vi "align_arrays.vi"(9 "IS_FRACTION":bool, 10 "Array 2":u8[](array[numeric]), 11 "Array":u8[](array[numeric])) -> (2 "Array 4":u8[](array[numeric]), 3 "Array 3":u8[](array[numeric]))   [LabVIEW 2025]
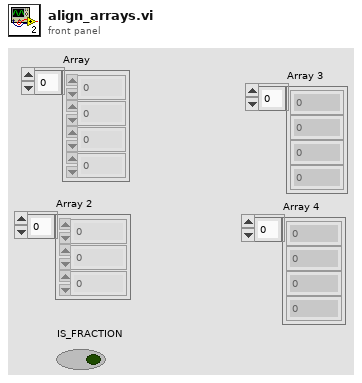
[diagram p1: front panel]
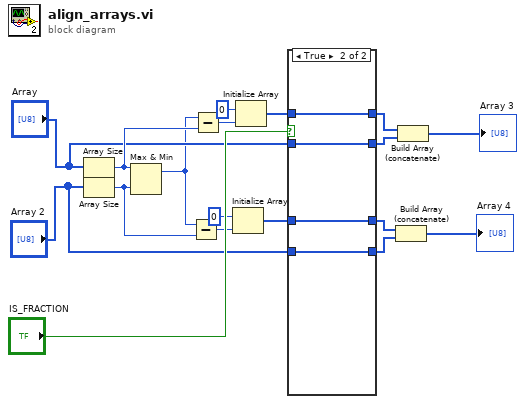
[diagram p0: block diagram]
diagram:
  n1 = Array Size(array="Array") -> (size(s)=w18:i32)
  n2 = Array Size(array="Array 2") -> (size(s)=w7:i32)
  n3 = Max & Min(x=w18, y=w7) -> (max(x,y)=w8:i32)  [unwired: 1 out]
  n4 = Subtract(x=w8, y=w7) -> (x-y=w6:i32)
  n5 = Subtract(x=w8, y=w18) -> (x-y=w17:i32)
  n6 = Initialize Array(u8 0 ("element"), w6) -> (w5:u8[])
  n7 = Initialize Array(u8 0 ("element"), w17) -> (w14:u8[])
  n8 = case shown="True" "IS_FRACTION" {
    tunnel: w14 -> [w21 w26]
    tunnel: [w22 w26] -> w12
    tunnel: "Array" -> [w22 w25]
    tunnel: [w21 w25] -> w11
    tunnel: w5 -> [w20 w24]
    tunnel: "Array 2" -> [w19 w23]
    tunnel: [w19 w24] -> w3
    tunnel: [w20 w23] -> w2
    frame False {
    }
    frame True {
    }
  }
  n9 = Build Array (concatenate)(w3, w2) -> (→"Array 4":u8[])
  n10 = Build Array (concatenate)(w12, w11) -> (→"Array 3":u8[])
